vi "SavePointCloudData.vi"(7 "handle":u64, 8 "error in (no error)":errorcluster caption="错误输入（无错误）", 9 "pstPointDataParam In":T1, 10 "pDstBuffer In":u8[](array[numeric]), 11 "pSrcData":u8[](array[numeric])) -> (0 "error out":errorcluster caption="错误输出", 1 "pstPointDataParam In":T1, 2 "pDstBuffer Out":u8[](array[numeric]), 3 "function return":i32, 5 "handle out":u64)   [LabVIEW 2011, in "MvCameraControl.lvlib"]
doc: "MV_LV_API int __stdcall SaveImage(MV_SAVE_IMAGE_PARAM* pSaveParam);"
uses:
  MvCameraControl.lvlib
  x86/MvCameraPatch.dll
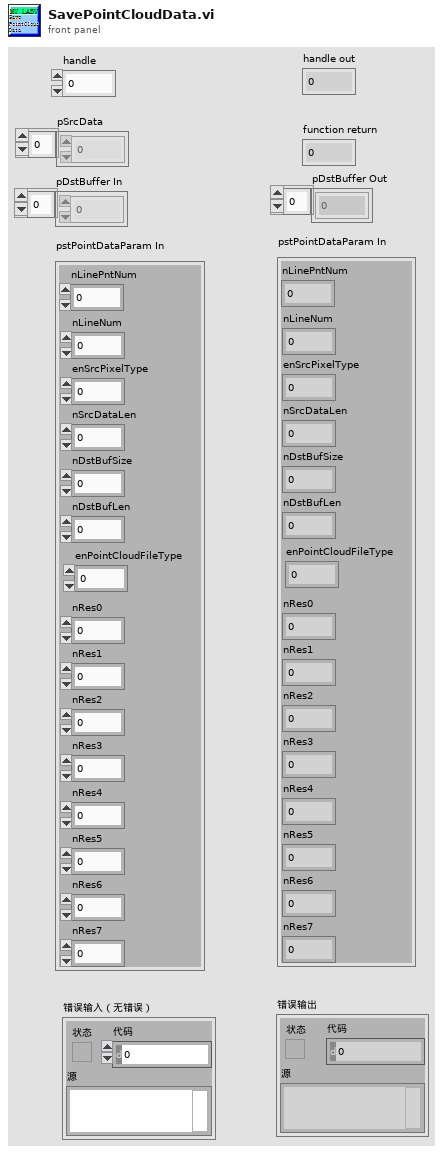
[diagram p1: front panel]
types:
  T1 = cluster{"nLineNum":u32, "enSrcPixelType":i32, "nSrcDataLen":u16, "nDstBufSize":u16, "nDstBufLen":u32, "enPointCloudFileType":u32, "nRes0":u32, "nRes1":u32, "nRes2":u32, "nRes3":u32, "nLinePntNum":u32, "nRes7":u32, "nRes6":u32, "nRes5":u32, "nRes4":u32}
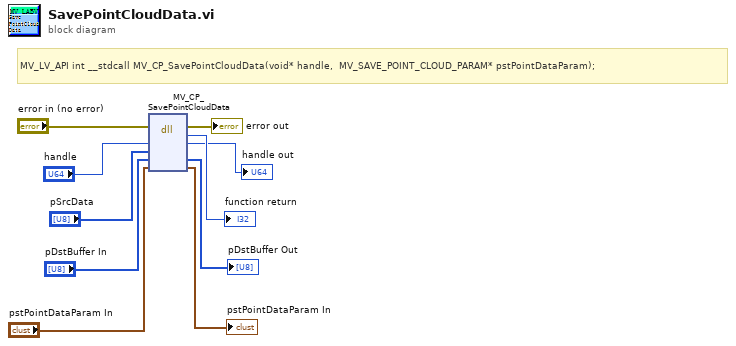
[diagram p0: block diagram]
diagram:
  # "MV_LV_API int __stdcall MV_CP_SavePointCloudData(void* handle,  MV_SAVE_POINT_CLOUD_PARAM* pstPointDataParam);"
  n1 = dll-call lib="F:/SVN/SDK/Release/MVS/Samples/Labview/MvLVLib/x86/MvCameraPatch.dll" fn="MV_CP_SavePointCloudData"(error in="error in (no error)", "handle"="handle", "pSrcData"="pSrcData", "pDstBuffer"="pDstBuffer In", "pstPointDataParam"="pstPointDataParam In") -> (error out=→"error out":errorcluster, "返回类型"=→"function return":i32, "handle"=→"handle out":u64, "pDstBuffer"=→"pDstBuffer Out":u8[], "pstPointDataParam"=→"pstPointDataParam In":T1)  [unwired: 3 in, 1 out]
